vi "Add New Or Old Label.vi"(8 "old label?":bool, 9 "refresh listbox":T6[](array[typedef]), 10 "label":T1) -> (1 "refresh listbox out":T6[](array[typedef]))   [LabVIEW 2020, in "AIM ARINC 429 System Explorer.lvlib" / "Implementation.lvlib"]
uses:
  Implementation.lvlib
  Types/Refresh Symbols.ctl
  Refresh Constants.vi
  <vilib>/NI/NI VeriStand Encoding and Decoding/Encoding.ctl
  <vilib>/NI/NI VeriStand Encoding and Decoding/Encoding and Decoding.lvlib
  Shared/Parameter Definition.ctl
  Shared/VS Channel Definition for Parameter.ctl
  Shared/Transfer Type.ctl
  Shared/VS Channels Definition for Label.ctl
  Types/Refresh Listbox.ctl
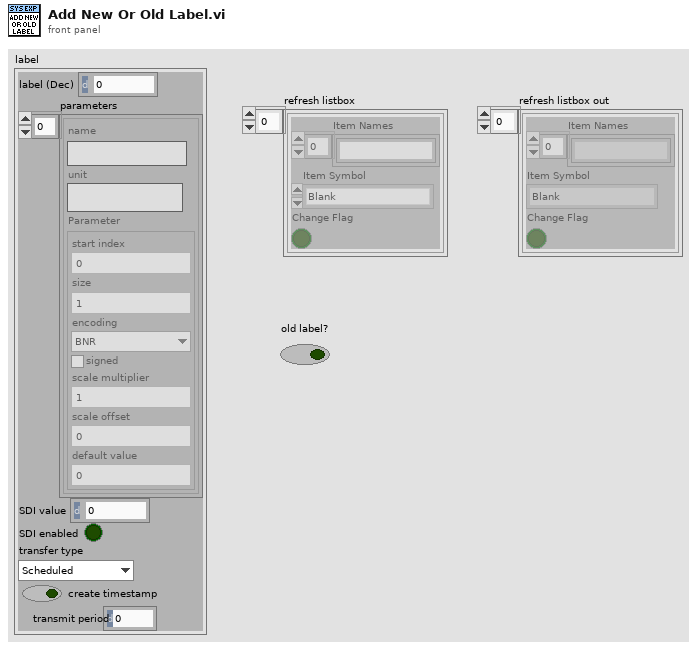
[diagram p1: front panel]
types:
  T1 = typedef "VS Channels Definition for Label.ctl" = cluster{"label (Dec)":u32, "parameters":T2[], "SDI value":u8, "SDI enabled":bool, "transfer type":T5, "create timestamp":bool, "transmit period":u32}
  T2 = typedef "VS Channel Definition for Parameter.ctl" = cluster{"name":string, "unit":string, "Parameter":T3}
  T3 = typedef "Parameter Definition.ctl" = cluster{"start index":i32, "size":i32, "encoding":T4, "signed":bool, "scale multiplier":dbl, "scale offset":dbl, "default value":dbl}
  T4 = typedef "Encoding and Decoding.lvlib/Encoding.ctl" = enum16{"BNR", "BCD", "Discrete"}
  T5 = typedef "Transfer Type.ctl" = enum16{"Scheduled", "Acyclic", "Block", "Strobe"}
  T6 = typedef "AIM ARINC 429 System Explorer.lvlib/Implementation.lvlib/Refresh Listbox.ctl" = cluster{"Item Names":string[], "Item Symbol":T7, "Change Flag":bool}
  T7 = typedef "AIM ARINC 429 System Explorer.lvlib/Implementation.lvlib/Refresh Symbols.ctl" = enum16{"Blank", "Port", "Incoming", "Outgoing", "Label", "Word", "Parameter", "ARINC-429", "Config Files", "Channel Spec", "Item"}
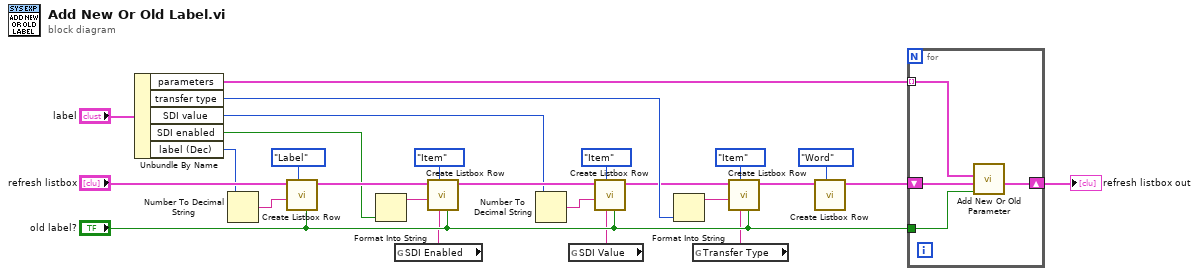
[diagram p0: block diagram]
diagram:
  n1 = Unbundle By Name("label") -> ("parameters"=w10:T2[], "transfer type"=w12:T5, "SDI value"=w16:u8, "SDI enabled"=w2:bool, "label (Dec)"=w21:u32)
  n2 = Number To Decimal String(number=w21) -> (decimal integer string=w23:string)  [unwired: 1 in]
  n3 = call "Create Listbox Row.vi"("swap new and old (F)"="old label?", "refresh symbol (Blank)"=Refresh_Symbols."Label" ("Refresh Symbol (Blank)"), "new item"=w23, "refresh listbox"="refresh listbox") -> ("refresh listbox out"=w19:T6[])  [unwired: 7 in]
  n4 = Format Into String(w2) -> (resulting string=w1:string)  [unwired: 3 in, 1 out]
  n5 = global read "Refresh Constants.vi" "SDI Enabled"() -> (w5:string)
  n6 = call "Create Listbox Row.vi"("swap new and old (F)"="old label?", "override name"=w5, "refresh symbol (Blank)"=Refresh_Symbols."Item" ("Refresh Symbol (Blank)"), "new item"=w1, "refresh listbox"=w19) -> ("refresh listbox out"=w17:T6[])  [unwired: 6 in]
  n7 = Number To Decimal String(number=w16) -> (decimal integer string=w18:string)  [unwired: 1 in]
  n8 = global read "Refresh Constants.vi" "SDI Value"() -> (w4:string)
  n9 = call "Create Listbox Row.vi"("swap new and old (F)"="old label?", "override name"=w4, "refresh symbol (Blank)"=Refresh_Symbols."Item" ("Refresh Symbol (Blank)"), "new item"=w18, "refresh listbox"=w17) -> ("refresh listbox out"=w11:T6[])  [unwired: 6 in]
  n10 = Format Into String(w12) -> (resulting string=w13:string)  [unwired: 3 in, 1 out]
  n11 = global read "Refresh Constants.vi" "Transfer Type"() -> (w3:string)
  n12 = call "Create Listbox Row.vi"("swap new and old (F)"="old label?", "override name"=w3, "refresh symbol (Blank)"=Refresh_Symbols."Item" ("Refresh Symbol (Blank)"), "new item"=w13, "refresh listbox"=w11) -> ("refresh listbox out"=w8:T6[])  [unwired: 6 in]
  n13 = call "Create Listbox Row.vi"("refresh symbol (Blank)"=Refresh_Symbols."Word" ("Refresh Symbol (Blank)"), "refresh listbox"=w8) -> ("refresh listbox out"=w7:T6[])  [unwired: 9 in]
  n14 = for {
    shift-right: [w27] -> w24
    shift-left: w7 -> [w30]
    tunnel: w10 -> [w28] mode=indexing
    tunnel: "old label?" -> [w29]
    n15 = call "Add New Or Old Parameter.vi"("old port?"=w29, "refresh listbox"=w30, "channel parameter"=w28) -> ("refresh listbox out"=w27:T6[])  [unwired: 8 in]
  }
  "refresh listbox out" <- w24
